vi "MakeHeader.vi"(7 "Header In":T1={"header info"={"Header"="", "Head length"=0}, "A/D info"={"# rf points per line"=0, "# lines per scan"=0, "sample rate MHz"=0, "# A/D bits"=0, "# bytes per A/D"=0, "TGC Flag"=0, "A/D Type"=""}, "Tranducer Info"={"bandwidth"=0.0, "center freq"=0.0, "start freq"=0.0, "ID"=0}, "Scan Info"={"delay"=0.0, "pivot distance"=0.0, "sector scan angle"=0.0, "operator"="", "Scan Mode"="", "location"=""}, "Time/Date Info"={"date"="", "time"=""}, "RF Info"={"RF file name"="", "RF file att"="", "RF cal file name"="", "RF cal file att"=""}, "Patient Info"={"ID"="", "extended ID"="", "age"=0, "sex"="", "previously\nscanned"="", "PSA"=0.0, "LOS"=1, "Ethnicty 2"=3, "Race"=3}, "Tissue Type"={"organ"=0, "disease type"=0, "disease location"=0, "IQ_pts"=0, "RcvBuffer"=0, "RcvFrame"=0, "IQBuff"=0, "IQFrame"=0, "IQPage"=0}, "Votage scaling"={"Digitizer (dB)"=0.0, "Gain (dB)"=0.0, "Atten (dB)"=0.0}, "Comment"="", "Misc Info"={"avg num"=0, "c speed"=0, "Div By or SF zones"=0, "XMIT CHS"=0, "RCV CHS"=0, "Xmit angle"=0.0}, "Therapy Parameters"={"Theraputic Freq (MHz)"=0.0, "Time on (s)"=0.0, "Therapy amplitude (mV)"=0.0, "Lines Before"=0, "Lines After"=0}, "Scan Settings"={"Energy (uJ or V)"=0, "Damp (Ohm) or Fc"=0, "HP Filt (KHz)"=0, "LP Filt (MHz)"=0, "Gain (db)"=0, "prf (kHz)"=0.0, "Distance between\nscan lines (um)"=0, "Distance between\nscan planes (um)"=0, "Scan line gap (um)"=0.0, "Scan plane gap (um)"=0.0}, "Compression Parameters"={"F1 (MHz)"=0.0, "F2 (MHz)"=0.0, "% taper"=0.0, "duration"=0.0}, "Patient Info Xtra"={"First Name"="", "Last Name"="", "Notes"=""}, "ROI Box"=[0, 0, 0, 0]} {"Compression Parameters"."% taper" min=50 max=1000 format="%.2f"; "Compression Parameters"."F2 (MHz)" format="%.3f"; "Compression Parameters"."F1 (MHz)" format="%.3f"; "Scan Settings"."prf (kHz)" format="%.2f"; "Therapy Parameters"."Therapy amplitude (mV)" min=50 max=1000 format="%.2f"; "Therapy Parameters"."Time on (s)" format="%.3f"; "Therapy Parameters"."Theraputic Freq (MHz)" format="%.3f"; "Patient Info"."Race" items=["Am Ind or Alaska", "Asian", "Hawaiian, Pac Isl", "Black or Afr Amer", "White", "more than one race", "unknown"]; "Patient Info"."Ethnicty 2" items=["Hispanic", "Non-Hispanic", "unknown"]; "Patient Info"."LOS" items=["1", "2", "3", "4", "5"]; "Patient Info"."PSA" format="%.1f"; "Scan Info"."delay" format="%.2f"; "Scan Info"."pivot distance" format="%.2f"; "Scan Info"."sector scan angle" format="%.2f"; "Tranducer Info"."bandwidth" format="%.2f"; "Tranducer Info"."center freq" format="%.2f"; "Tranducer Info"."start freq" format="%.2f"}) -> (3 "Header String":string)   [LabVIEW 2022 SP3]
uses:
  Header.ctl
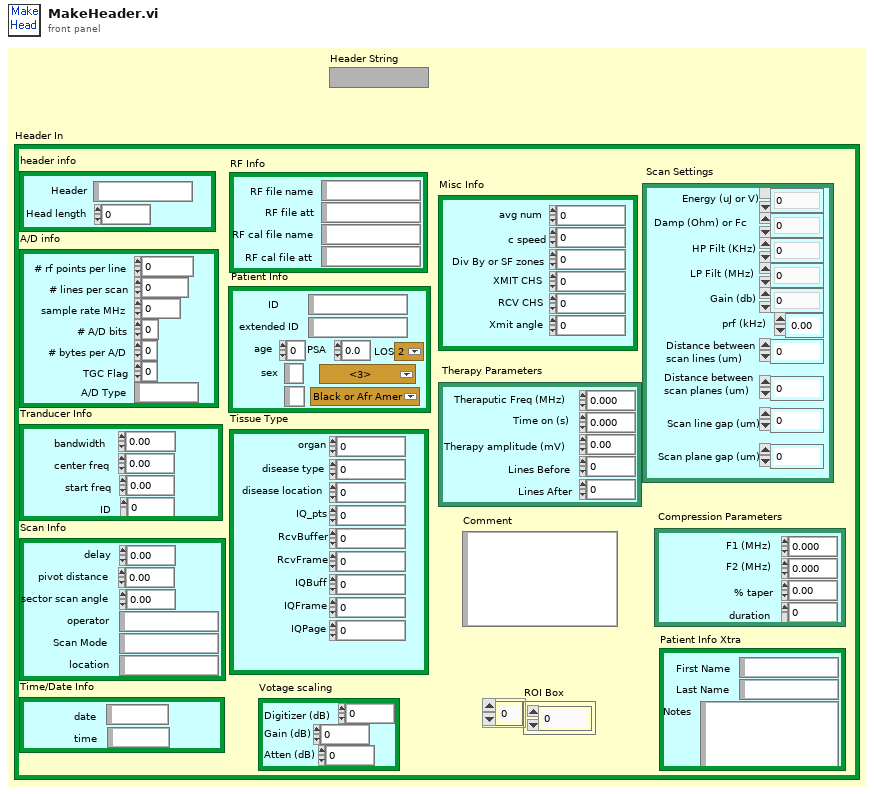
[diagram p1: front panel]
types:
  T1 = typedef "Header.ctl" = cluster{"header info":cluster{"Header":string, "Head length":i16}, "A/D info":cluster{"# rf points per line":u16, "# lines per scan":u16, "sample rate MHz":u16, "# A/D bits":i16, "# bytes per A/D":u16, "TGC Flag":u16, "A/D Type":string}, "Tranducer Info":cluster{"bandwidth":sgl, "center freq":sgl, "start freq":sgl, "ID":i32}, "Scan Info":cluster{"delay":sgl, "pivot distance":sgl, "sector scan angle":sgl, "operator":string, "Scan Mode":string, "location":string}, "Time/Date Info":cluster{"date":string, "time":string}, "RF Info":cluster{"RF file name":string, "RF file att":string, "RF cal file name":string, "RF cal file att":string}, "Patient Info":cluster{"ID":string, "extended ID":string, "age":u16, "sex":string, "previously\nscanned":string, "PSA":sgl, "LOS":u8, "Ethnicty 2":u8, "Race":u8}, "Tissue Type":cluster{"organ":i16, "disease type":i16, "disease location":i16, "IQ_pts":u16, "RcvBuffer":u8, "RcvFrame":u16, "IQBuff":u8, "IQFrame":u16, "IQPage":u8}, "Votage scaling":cluster{"Digitizer (dB)":sgl, "Gain (dB)":sgl, "Atten (dB)":sgl}, "Comment":string, "Misc Info":cluster{"avg num":u16, "c speed":i16, "Div By or SF zones":i16, "XMIT CHS":u8, "RCV CHS":u8, "Xmit angle":sgl}, "Therapy Parameters":cluster{"Theraputic Freq (MHz)":sgl, "Time on (s)":sgl, "Therapy amplitude (mV)":sgl, "Lines Before":u16, "Lines After":u16}, "Scan Settings":cluster{"Energy (uJ or V)":u8, "Damp (Ohm) or Fc":u8, "HP Filt (KHz)":u8, "LP Filt (MHz)":u8, "Gain (db)":u8, "prf (kHz)":sgl, "Distance between\nscan lines (um)":u16, "Distance between\nscan planes (um)":u16, "Scan line gap (um)":sgl, "Scan plane gap (um)":sgl}, "Compression Parameters":cluster{"F1 (MHz)":sgl, "F2 (MHz)":sgl, "% taper":sgl, "duration":sgl}, "Patient Info Xtra":cluster{"First Name":string, "Last Name":string, "Notes":string}, "ROI Box":u16[]}
  T2 = cluster{"# rf points per line":u16, "# lines per scan":u16, "sample rate MHz":u16, "# A/D bits":i16, "# bytes per A/D":u16, "TGC Flag":u16, "A/D Type":string}
  T3 = cluster{"bandwidth":sgl, "center freq":sgl, "start freq":sgl, "ID":i32}
  T4 = cluster{"delay":sgl, "pivot distance":sgl, "sector scan angle":sgl, "operator":string, "Scan Mode":string, "location":string}
  T5 = cluster{"RF file name":string, "RF file att":string, "RF cal file name":string, "RF cal file att":string}
  T6 = cluster{"ID":string, "extended ID":string, "age":u16, "sex":string, "previously\nscanned":string, "PSA":sgl, "LOS":u8, "Ethnicty 2":u8, "Race":u8}
  T7 = cluster{"organ":i16, "disease type":i16, "disease location":i16, "IQ_pts":u16, "RcvBuffer":u8, "RcvFrame":u16, "IQBuff":u8, "IQFrame":u16, "IQPage":u8}
  T8 = cluster{"Digitizer (dB)":sgl, "Gain (dB)":sgl, "Atten (dB)":sgl}
  T9 = cluster{"avg num":u16, "c speed":i16, "Div By or SF zones":i16, "XMIT CHS":u8, "RCV CHS":u8, "Xmit angle":sgl}
  T10 = cluster{"Theraputic Freq (MHz)":sgl, "Time on (s)":sgl, "Therapy amplitude (mV)":sgl, "Lines Before":u16, "Lines After":u16}
  T11 = cluster{"Energy (uJ or V)":u8, "Damp (Ohm) or Fc":u8, "HP Filt (KHz)":u8, "LP Filt (MHz)":u8, "Gain (db)":u8, "prf (kHz)":sgl, "Distance between\nscan lines (um)":u16, "Distance between\nscan planes (um)":u16, "Scan line gap (um)":sgl, "Scan plane gap (um)":sgl}
  T12 = cluster{"F1 (MHz)":sgl, "F2 (MHz)":sgl, "% taper":sgl, "duration":sgl}
  T13 = cluster{"First Name":string, "Last Name":string, "Notes":string}
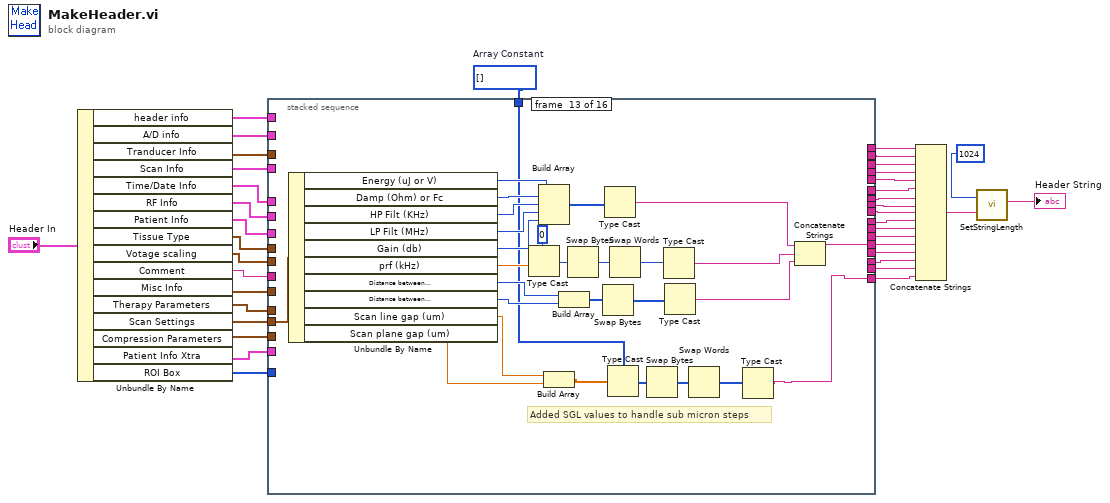
[diagram p0: block diagram]
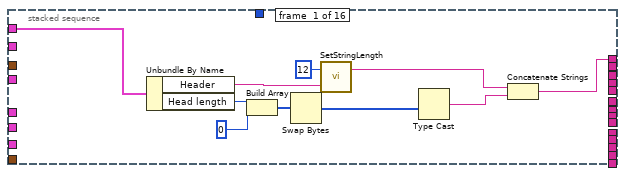
[diagram p2: hidden frame]
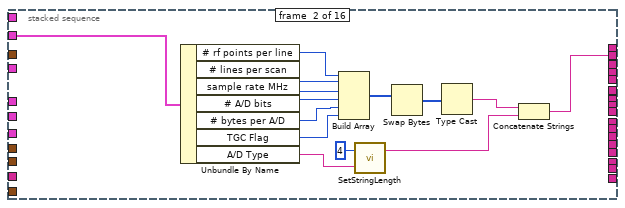
[diagram p3: hidden frame]
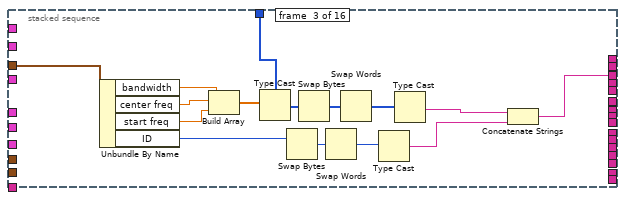
[diagram p4: hidden frame]
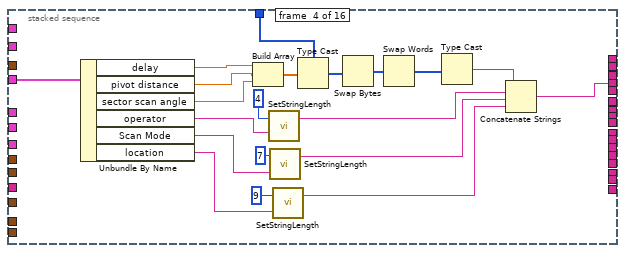
[diagram p5: hidden frame]
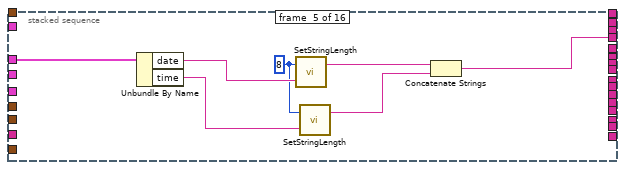
[diagram p6: hidden frame]
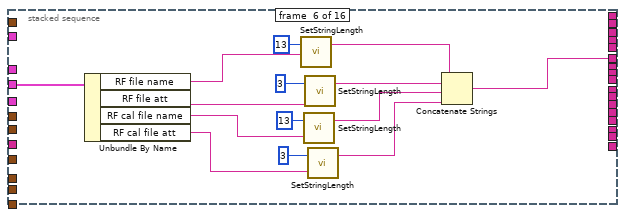
[diagram p7: hidden frame]
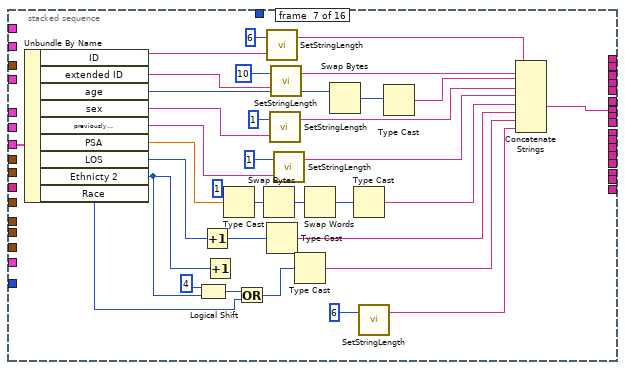
[diagram p8: hidden frame]
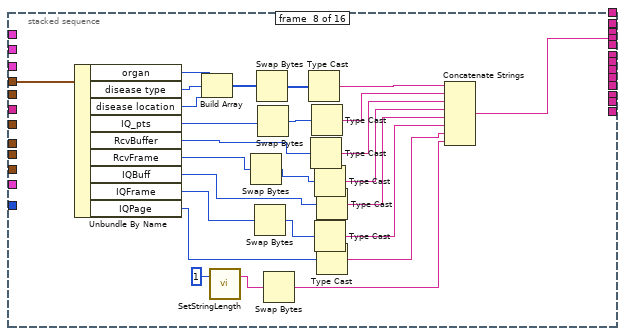
[diagram p9: hidden frame]
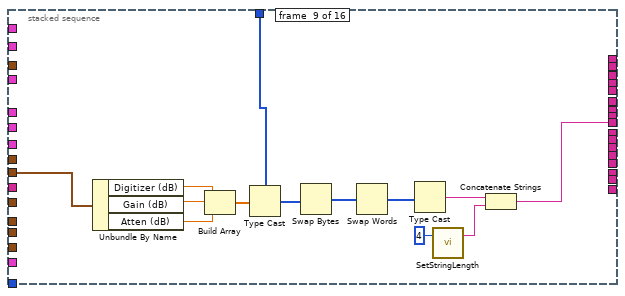
[diagram p10: hidden frame]
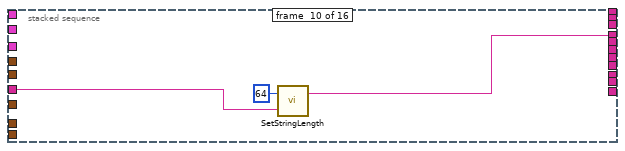
[diagram p11: hidden frame]
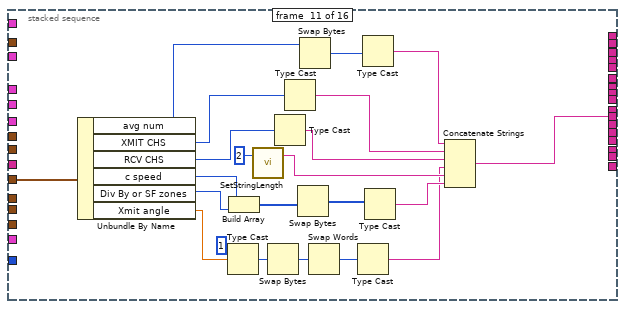
[diagram p12: hidden frame]
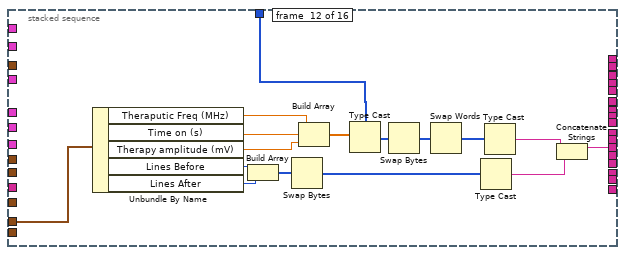
[diagram p13: hidden frame]
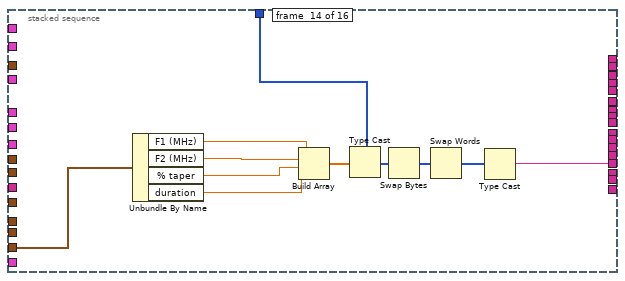
[diagram p14: hidden frame]
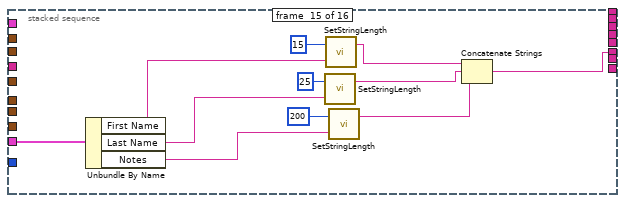
[diagram p15: hidden frame]
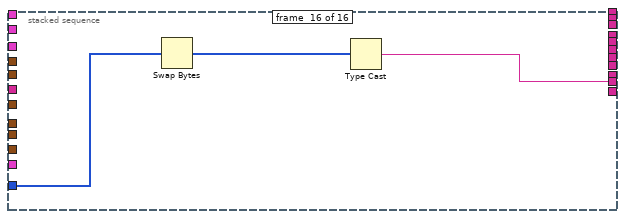
[diagram p16: hidden frame]
diagram:
  w38 = i32[] []  # Array Constant
  n1 = Unbundle By Name("Header In") -> ("header info"=w37:cluster{"Header":string, "Head length":i16}, "A/D info"=w34:T2, "Tranducer Info"=w32:T3, "Scan Info"=w30:T4, "Time/Date Info"=w15:cluster{"date":string, "time":string}, "RF Info"=w14:T5, "Patient Info"=w13:T6, "Tissue Type"=w12:T7, "Votage scaling"=w10:T8, "Comment"=w9:string, "Misc Info"=w22:T9, "Therapy Parameters"=w8:T10, "Scan Settings"=w36:T11, "Compression Parameters"=w16:T12, "Patient Info Xtra"=w11:T13, "ROI Box"=w7:u16[])
  n2 = stacked-sequence {
    tunnel: w37 -> [w40 _ _ _ _ _ _ _ _ _ _ _ _ _ _ _]
    tunnel: [w39 _ _ _ _ _ _ _ _ _ _ _ _ _ _ _] -> w35
    tunnel: w34 -> [_ w51 _ _ _ _ _ _ _ _ _ _ _ _ _ _]
    tunnel: [_ w50 _ _ _ _ _ _ _ _ _ _ _ _ _ _] -> w33
    tunnel: w32 -> [_ _ w66 _ _ _ _ _ _ _ _ _ _ _ _ _]
    tunnel: [_ _ w65 _ _ _ _ _ _ _ _ _ _ _ _ _] -> w31
    tunnel: w38 -> [_ _ w64 w78 _ _ _ _ w180 _ _ w221 w234 w264 _ _]
    tunnel: w30 -> [_ _ _ w80 _ _ _ _ _ _ _ _ _ _ _ _]
    tunnel: [_ _ _ w79 _ _ _ _ _ _ _ _ _ _ _ _] -> w29
    tunnel: w15 -> [_ _ _ _ w99 _ _ _ _ _ _ _ _ _ _ _]
    tunnel: [_ _ _ _ w98 _ _ _ _ _ _ _ _ _ _ _] -> w28
    tunnel: w14 -> [_ _ _ _ _ w106 _ _ _ _ _ _ _ _ _ _]
    tunnel: [_ _ _ _ _ w105 _ _ _ _ _ _ _ _ _ _] -> w27
    tunnel: w13 -> [_ _ _ _ _ _ w126 _ _ _ _ _ _ _ _ _]
    tunnel: [_ _ _ _ _ _ w125 _ _ _ _ _ _ _ _ _] -> w26
    tunnel: w12 -> [_ _ _ _ _ _ _ w171 _ _ _ _ _ _ _ _]
    tunnel: [_ _ _ _ _ _ _ w170 _ _ _ _ _ _ _ _] -> w25
    tunnel: w10 -> [_ _ _ _ _ _ _ _ w189 _ _ _ _ _ _ _]
    tunnel: [_ _ _ _ _ _ _ _ w188 _ _ _ _ _ _ _] -> w24
    tunnel: w9 -> [_ _ _ _ _ _ _ _ _ w193 _ _ _ _ _ _]
    tunnel: [_ _ _ _ _ _ _ _ _ w192 _ _ _ _ _ _] -> w23
    tunnel: w22 -> [_ _ _ _ _ _ _ _ _ _ w209 _ _ _ _ _]
    tunnel: [_ _ _ _ _ _ _ _ _ _ w208 _ _ _ _ _] -> w21
    tunnel: w8 -> [_ _ _ _ _ _ _ _ _ _ _ w220 _ _ _ _]
    tunnel: [_ _ _ _ _ _ _ _ _ _ _ w219 _ _ _ _] -> w18
    tunnel: w36 -> [_ _ _ _ _ _ _ _ _ _ _ _ w243 _ _ _]
    tunnel: [_ _ _ _ _ _ _ _ _ _ _ _ w242 _ _ _] -> w20
    tunnel: [_ _ _ _ _ _ _ _ _ _ _ _ _ w261 _ _] -> w19
    tunnel: [_ _ _ _ _ _ _ _ _ _ _ _ _ _ w272 _] -> w17
    tunnel: w16 -> [_ _ _ _ _ _ _ _ _ _ _ _ _ w262 _ _]
    tunnel: w11 -> [_ _ _ _ _ _ _ _ _ _ _ _ _ _ w279 _]
    tunnel: w7 -> [_ _ _ _ _ _ _ _ _ _ _ _ _ _ _ w283]
    tunnel: [_ _ _ _ _ _ _ _ _ _ _ _ _ _ _ w284] -> w3
    tunnel: [_ _ _ _ _ _ _ _ _ _ _ _ w233 _ _ _] -> w1
    frame #0 {
      n3 = Unbundle By Name(w40) -> ("Header"=w41:string, "Head length"=w43:i16)
      n4 = Build Array(w43, i16 0) -> (w45:i16[])
      n5 = Swap Bytes(anything=w45) -> (byte swapped=w47:i16[])
      n6 = call "SetStringLength.vi"("Input String"=w41, "String Length"=12) -> ("Output String"=w46:string)  [unwired: 1 out]
      n7 = Type Cast(x=w47) -> (*(type *) &x=w48:string)  [unwired: 1 out]
      n8 = Concatenate Strings(w46, w48) -> (w39:string)
    }
    frame #1 {
      n9 = Unbundle By Name(w51) -> ("# rf points per line"=w52:u16, "# lines per scan"=w53:u16, "sample rate MHz"=w54:u16, "# A/D bits"=w55:i16, "# bytes per A/D"=w61:u16, "TGC Flag"=w62:u16, "A/D Type"=w49:string)
      n10 = Build Array(w52, w53, w54, w55, w61, w62) -> (w56:u16[])
      n11 = call "SetStringLength.vi"("Input String"=w49, "String Length"=4) -> ("Output String"=w59:string)  [unwired: 1 out]
      n12 = Swap Bytes(anything=w56) -> (byte swapped=w58:u16[])
      n13 = Type Cast(x=w58) -> (*(type *) &x=w60:string)  [unwired: 1 out]
      n14 = Concatenate Strings(w60, w59) -> (w50:string)
    }
    frame #2 {
      n15 = Unbundle By Name(w66) -> ("bandwidth"=w63:sgl, "center freq"=w68:sgl, "start freq"=w67:sgl, "ID"=w69:i32)
      n16 = Build Array(w63, w68, w67) -> (w74:sgl[])
      n17 = Type Cast(type=w64, x=w74) -> (*(type *) &x=w75:i32[])
      n18 = Swap Bytes(anything=w69) -> (byte swapped=w70:i32)
      n19 = Swap Bytes(anything=w75) -> (byte swapped=w71:i32[])
      n20 = Swap Words(1:w70) -> (0:w72:i32)
      n21 = Swap Words(1:w71) -> (0:w76:i32[])
      n22 = Type Cast(x=w72) -> (*(type *) &x=w73:string)  [unwired: 1 out]
      n23 = Type Cast(x=w76) -> (*(type *) &x=w77:string)  [unwired: 1 out]
      n24 = Concatenate Strings(w77, w73) -> (w65:string)
    }
    frame #3 {
      n25 = Unbundle By Name(w80) -> ("delay"=w87:sgl, "pivot distance"=w88:sgl, "sector scan angle"=w89:sgl, "operator"=w81:string, "Scan Mode"=w82:string, "location"=w83:string)
      n26 = Build Array(w87, w88, w89) -> (w94:sgl[])
      n27 = call "SetStringLength.vi"("Input String"=w81, "String Length"=4) -> ("Output String"=w91:string)  [unwired: 1 out]
      n28 = call "SetStringLength.vi"("Input String"=w82, "String Length"=7) -> ("Output String"=w92:string)  [unwired: 1 out]
      n29 = call "SetStringLength.vi"("Input String"=w83, "String Length"=9) -> ("Output String"=w93:string)  [unwired: 1 out]
      n30 = Type Cast(type=w78, x=w94) -> (*(type *) &x=w95:i32[])
      n31 = Swap Bytes(anything=w95) -> (byte swapped=w90:i32[])
      n32 = Swap Words(1:w90) -> (0:w96:i32[])
      n33 = Type Cast(x=w96) -> (*(type *) &x=w97:string)  [unwired: 1 out]
      n34 = Concatenate Strings(w97, w91, w92, w93) -> (w79:string)
    }
    frame #4 {
      w100 = 8 ("String Length")
      n35 = Unbundle By Name(w99) -> ("date"=w101:string, "time"=w102:string)
      n36 = call "SetStringLength.vi"("Input String"=w101, "String Length"=w100) -> ("Output String"=w103:string)  [unwired: 1 out]
      n37 = call "SetStringLength.vi"("Input String"=w102, "String Length"=w100) -> ("Output String"=w104:string)  [unwired: 1 out]
      n38 = Concatenate Strings(w103, w104) -> (w98:string)
    }
    frame #5 {
      n39 = Unbundle By Name(w106) -> ("RF file name"=w107:string, "RF file att"=w108:string, "RF cal file name"=w112:string, "RF cal file att"=w113:string)
      n40 = call "SetStringLength.vi"("Input String"=w107, "String Length"=13) -> ("Output String"=w115:string)  [unwired: 1 out]
      n41 = call "SetStringLength.vi"("Input String"=w112, "String Length"=13) -> ("Output String"=w117:string)  [unwired: 1 out]
      n42 = call "SetStringLength.vi"("Input String"=w108, "String Length"=3) -> ("Output String"=w116:string)  [unwired: 1 out]
      n43 = call "SetStringLength.vi"("Input String"=w113, "String Length"=3) -> ("Output String"=w118:string)  [unwired: 1 out]
      n44 = Concatenate Strings(w115, w116, w117, w118) -> (w105:string)
    }
    frame #6 {
      n45 = Unbundle By Name(w126) -> ("ID"=w132:string, "extended ID"=w133:string, "age"=w131:u16, "sex"=w134:string, "previously\nscanned"=w135:string, "PSA"=w144:sgl, "LOS"=w148:u8, "Ethnicty 2"=w121:u8, "Race"=w120:u8)
      n46 = Logical Shift(y=4, x=w121) -> (x << y=w123:u8)
      n47 = Increment(x=w148) -> (x+1=w151:u8)
      n48 = Increment(x=w121) -> ()  [unwired: 1 out]
      n49 = Type Cast(type=1 ("String Length"), x=w144) -> (*(type *) &x=w149:i32)
      n50 = Or(x=w123, y=w120) -> (x .or. y?=w122:u8)
      n51 = Swap Bytes(anything=w149) -> (byte swapped=w143:i32)
      n52 = call "SetStringLength.vi"("Input String"=w132, "String Length"=6) -> ("Output String"=w142:string)  [unwired: 1 out]
      n53 = Type Cast(x=w151) -> (*(type *) &x=w152:string)  [unwired: 1 out]
      n54 = call "SetStringLength.vi"("Input String"=w134, "String Length"=1) -> ("Output String"=w138:string)  [unwired: 1 out]
      n55 = call "SetStringLength.vi"("Input String"=w133, "String Length"=10) -> ("Output String"=w141:string)  [unwired: 1 out]
      n56 = call "SetStringLength.vi"("Input String"=w135, "String Length"=1) -> ("Output String"=w139:string)  [unwired: 1 out]
      n57 = Type Cast(x=w122) -> (*(type *) &x=w119:string)  [unwired: 1 out]
      n58 = Swap Words(1:w143) -> (0:w145:i32)
      n59 = Swap Bytes(anything=w131) -> (byte swapped=w136:u16)
      n60 = Type Cast(x=w145) -> (*(type *) &x=w147:string)  [unwired: 1 out]
      n61 = call "SetStringLength.vi"("String Length"=6) -> ("Output String"=w146:string)  [unwired: 1 in, 1 out]
      n62 = Type Cast(x=w136) -> (*(type *) &x=w137:string)  [unwired: 1 out]
      n63 = Concatenate Strings(w142, w141, w137, w138, w139, w147, w152, w119, w146) -> (w125:string)
    }
    frame #7 {
      n64 = Unbundle By Name(w171) -> ("organ"=w172:i16, "disease type"=w173:i16, "disease location"=w174:i16, "IQ_pts"=w169:u16, "RcvBuffer"=w166:u8, "RcvFrame"=w165:u16, "IQBuff"=w163:u8, "IQFrame"=w159:u16, "IQPage"=w157:u8)
      n65 = Build Array(w172, w173, w174) -> (w176:i16[])
      n66 = call "SetStringLength.vi"("String Length"=1) -> ("Output String"=w154:string)  [unwired: 1 in, 1 out]
      n67 = Swap Bytes(anything=w165) -> (byte swapped=w164:u16)
      n68 = Swap Bytes(anything=w159) -> (byte swapped=w158:u16)
      n69 = Swap Bytes(anything=w176) -> (byte swapped=w175:i16[])
      n70 = Swap Bytes(anything=w169) -> (byte swapped=w168:u16)
      n71 = Swap Bytes(anything=w154) -> (byte swapped=w153:string)
      n72 = Type Cast(x=w175) -> (*(type *) &x=w178:string)  [unwired: 1 out]
      n73 = Type Cast(x=w166) -> (*(type *) &x=w162:string)  [unwired: 1 out]
      n74 = Type Cast(x=w168) -> (*(type *) &x=w167:string)  [unwired: 1 out]
      n75 = Type Cast(x=w164) -> (*(type *) &x=w161:string)  [unwired: 1 out]
      n76 = Type Cast(x=w158) -> (*(type *) &x=w156:string)  [unwired: 1 out]
      n77 = Type Cast(x=w163) -> (*(type *) &x=w160:string)  [unwired: 1 out]
      n78 = Type Cast(x=w157) -> (*(type *) &x=w155:string)  [unwired: 1 out]
      n79 = Concatenate Strings(w178, w167, w162, w161, w160, w156, w155, w153) -> (w170:string)
    }
    frame #8 {
      n80 = Unbundle By Name(w189) -> ("Digitizer (dB)"=w183:sgl, "Gain (dB)"=w182:sgl, "Atten (dB)"=w181:sgl)
      n81 = Build Array(w183, w182, w181) -> (w185:sgl[])
      n82 = Type Cast(type=w180, x=w185) -> (*(type *) &x=w186:i32[])
      n83 = Swap Bytes(anything=w186) -> (byte swapped=w184:i32[])
      n84 = Swap Words(1:w184) -> (0:w187:i32[])
      n85 = Type Cast(x=w187) -> (*(type *) &x=w179:string)  [unwired: 1 out]
      n86 = call "SetStringLength.vi"("String Length"=4) -> ("Output String"=w191:string)  [unwired: 1 in, 1 out]
      n87 = Concatenate Strings(w179, w191) -> (w188:string)
    }
    frame #9 {
      n88 = call "SetStringLength.vi"("Input String"=w193, "String Length"=64) -> ("Output String"=w192:string)  [unwired: 1 out]
    }
    frame #10 {
      n89 = Unbundle By Name(w209) -> ("avg num"=w207:u16, "XMIT CHS"=w206:u8, "RCV CHS"=w205:u8, "c speed"=w216:i16, "Div By or SF zones"=w215:i16, "Xmit angle"=w197:sgl)
      n90 = Type Cast(type=1 ("String Length"), x=w197) -> (*(type *) &x=w200:i32)
      n91 = Build Array(w216, w215) -> (w210:i16[])
      n92 = call "SetStringLength.vi"("String Length"=2) -> ("Output String"=w214:string)  [unwired: 1 in, 1 out]
      n93 = Swap Bytes(anything=w200) -> (byte swapped=w198:i32)
      n94 = Type Cast(x=w205) -> (*(type *) &x=w202:string)  [unwired: 1 out]
      n95 = Type Cast(x=w206) -> (*(type *) &x=w203:string)  [unwired: 1 out]
      n96 = Swap Bytes(anything=w210) -> (byte swapped=w212:i16[])
      n97 = Swap Bytes(anything=w207) -> (byte swapped=w213:u16)
      n98 = Swap Words(1:w198) -> (0:w199:i32)
      n99 = Type Cast(x=w199) -> (*(type *) &x=w195:string)  [unwired: 1 out]
      n100 = Type Cast(x=w213) -> (*(type *) &x=w204:string)  [unwired: 1 out]
      n101 = Type Cast(x=w212) -> (*(type *) &x=w196:string)  [unwired: 1 out]
      n102 = Concatenate Strings(w204, w203, w202, w195, w214, w196) -> (w208:string)
    }
    frame #11 {
      n103 = Unbundle By Name(w220) -> ("Theraputic Freq (MHz)"=w226:sgl, "Time on (s)"=w227:sgl, "Therapy amplitude (mV)"=w228:sgl, "Lines Before"=w230:u16, "Lines After"=w231:u16)
      n104 = Build Array(w230, w231) -> (w229:u16[])
      n105 = Swap Bytes(anything=w229) -> (byte swapped=w232:u16[])
      n106 = Build Array(w226, w227, w228) -> (w223:sgl[])
      n107 = Type Cast(type=w221, x=w223) -> (*(type *) &x=w224:i32[])
      n108 = Swap Bytes(anything=w224) -> (byte swapped=w222:i32[])
      n109 = Swap Words(1:w222) -> (0:w225:i32[])
      n110 = Type Cast(x=w232) -> (*(type *) &x=w217:string)  [unwired: 1 out]
      n111 = Type Cast(x=w225) -> (*(type *) &x=w218:string)  [unwired: 1 out]
      n112 = Concatenate Strings(w218, w217) -> (w219:string)
    }
    frame #12 {
      # "Added SGL values to handle sub micron steps"
      n113 = Unbundle By Name(w243) -> ("Energy (uJ or V)"=w244:u8, "Damp (Ohm) or Fc"=w245:u8, "HP Filt (KHz)"=w246:u8, "LP Filt (MHz)"=w247:u8, "Gain (db)"=w248:u8, "prf (kHz)"=w253:sgl, "Distance between\nscan lines (um)"=w256:u16, "Distance between\nscan planes (um)"=w241:u16, "Scan line gap (um)"=w237:sgl, "Scan plane gap (um)"=w236:sgl)
      n114 = Type Cast(type=0, x=w253) -> (*(type *) &x=w251:i32)
      n115 = Build Array(w244, w245, w246, w247, w248) -> (w249:u8[])
      n116 = Build Array(w237, w236) -> (w235:sgl[])
      n117 = Build Array(w256, w241) -> (w255:u16[])
      n118 = Swap Bytes(anything=w251) -> (byte swapped=w250:i32)
      n119 = Swap Bytes(anything=w255) -> (byte swapped=w257:u16[])
      n120 = Type Cast(x=w249) -> (*(type *) &x=w258:string)  [unwired: 1 out]
      n121 = Type Cast(type=w234, x=w235) -> (*(type *) &x=w239:i32[])
      n122 = Swap Words(1:w250) -> (0:w252:i32)
      n123 = Swap Bytes(anything=w239) -> (byte swapped=w238:i32[])
      n124 = Type Cast(x=w252) -> (*(type *) &x=w259:string)  [unwired: 1 out]
      n125 = Type Cast(x=w257) -> (*(type *) &x=w260:string)  [unwired: 1 out]
      n126 = Swap Words(1:w238) -> (0:w240:i32[])
      n127 = Type Cast(x=w240) -> (*(type *) &x=w233:string)  [unwired: 1 out]
      n128 = Concatenate Strings(w258, w259, w260) -> (w242:string)
    }
    frame #13 {
      n129 = Unbundle By Name(w262) -> ("F1 (MHz)"=w269:sgl, "F2 (MHz)"=w270:sgl, "% taper"=w271:sgl, "duration"=w263:sgl)
      n130 = Build Array(w269, w270, w271, w263) -> (w266:sgl[])
      n131 = Type Cast(type=w264, x=w266) -> (*(type *) &x=w267:i32[])
      n132 = Swap Bytes(anything=w267) -> (byte swapped=w265:i32[])
      n133 = Swap Words(1:w265) -> (0:w268:i32[])
      n134 = Type Cast(x=w268) -> (*(type *) &x=w261:string)  [unwired: 1 out]
    }
    frame #14 {
      n135 = Unbundle By Name(w279) -> ("First Name"=w278:string, "Last Name"=w277:string, "Notes"=w276:string)
      n136 = call "SetStringLength.vi"("Input String"=w277, "String Length"=25) -> ("Output String"=w274:string)  [unwired: 1 out]
      n137 = call "SetStringLength.vi"("Input String"=w278, "String Length"=15) -> ("Output String"=w275:string)  [unwired: 1 out]
      n138 = call "SetStringLength.vi"("Input String"=w276, "String Length"=200) -> ("Output String"=w273:string)  [unwired: 1 out]
      n139 = Concatenate Strings(w275, w274, w273) -> (w272:string)
    }
    frame #15 {
      n140 = Swap Bytes(anything=w283) -> (byte swapped=w285:u16[])
      n141 = Type Cast(x=w285) -> (*(type *) &x=w284:string)  [unwired: 1 out]
    }
  }
  n142 = Concatenate Strings(w35, w33, w31, w29, w28, w27, w26, w25, w24, w23, w21, w18, w20, w19, w17, w3, w1) -> (w4:string)
  n143 = call "SetStringLength.vi"("Input String"=w4, "String Length"=1024) -> ("Output String"=→"Header String":string)  [unwired: 1 out]
